vi "Stop Core.vi"(10 "final error code":i32 caption="code d'erreur final", 11 "Water Level in":refnum<class "Water Level.lvclass"> caption="Acteur en entrée") -> (3 "Water Level out":refnum<class "Water Level.lvclass"> caption="Acteur en sortie")   [LabVIEW 2015, in "Water Level.lvclass"]
doc: "(<B>Nom de fichier</B> : Actor Framework.lvlib:Actor.lvclass:Stop Core.vi)\n\nDéfinit ce que l'acteur fait avant de s'arrêter. Utilisez l'entrée <B>code d'erreur final</B> pour déterminer si l'acteur se ferme en réponse à une erreur.\n\nPar défaut, cette méthode ne fait rien. Une classe descendante peut la redéfinir pour configurer un comportement, tel que la fermeture des processus initialisés par l'acteur dans sa redéfinition de la méthode Noyau d'acteur."
uses:
  Water Level.lvclass
  Simulation/Simulation Data_Global.vi
  Level Controller/Level Controller/Level Controller.lvclass
  Simulation/Simulation.lvlib
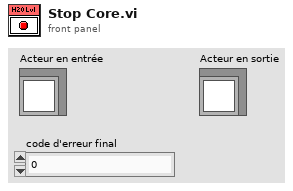
[diagram p1: front panel]
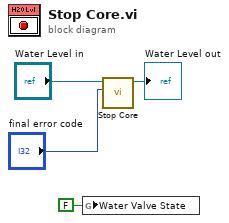
[diagram p0: block diagram]
diagram:
  n1 = global write "Simulation Data_Global.vi" "Water Valve State"(FALSE ("Water Valve State")) -> ()
  n2 = call-parent "Stop Core.vi"("final error code"="final error code", "Actor in"="Water Level in") -> ("Actor out"=→"Water Level out":refnum<class "Water Level.lvclass">)  [unwired: 9 in]
